vi "Shift_Register_drivingstepperMotor.vi"() -> ()   [LabVIEW 2015]
panel:
  in  "stop":bool
  in  "millisecond multiple":u32
  out "appended array":i32[](array[numeric]) format="%b"
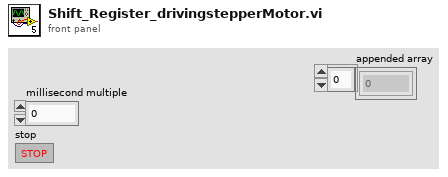
[diagram p1: front panel]
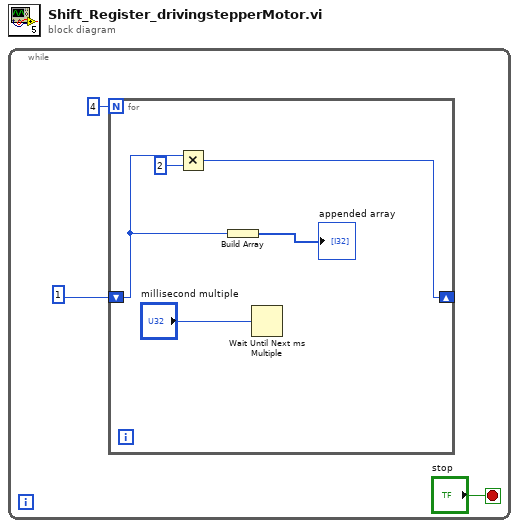
[diagram p0: block diagram]
diagram:
  n1 = while {
    stop <- "stop" stop-if-true
    n2 = for {
      N: 4 -> [_]
      shift-right: [w8] -> _
      shift-left: 1 -> [w6]
      n3 = Multiply(x=w6, y=i8 2) -> (x*y=w8:i32)
      n4 = Build Array(w6) -> (→"appended array":i32[])
      n5 = Wait Until Next ms Multiple(millisecond multiple="millisecond multiple") -> ()  [unwired: 1 out]
    }
  }
